vi "Divide Sweep Config by Output Gain.vi"(8 "error in (no error)":errorcluster, 11 "Instrument.DAQ":refnum<class "Instrument.DAQ.lvclass">) -> (0 "error out":errorcluster, 3 "Instrument.DAQ out":refnum<class "Instrument.DAQ.lvclass">)   [LabVIEW 2019, in "Instrument.Lockin.lvlib" / "Instrument.DAQ.lvclass"]
uses:
  Instrument.DAQ.lvclass
  Instrument.DAQ.lvclass/Instrument.DAQ.ctl
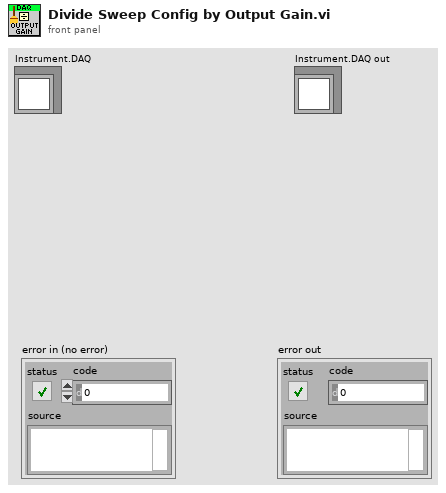
[diagram p1: front panel]
types:
  T1 = typedef "Instrument.Lockin.lvlib/Instrument.DAQ.lvclass/Sweep.Channel--Cluster--Array.ctl" = T2[]
  T2 = typedef "Instrument.Lockin.lvlib/Instrument.DAQ.lvclass/Sweep.Channel--Cluster.ctl" = cluster{"Enable?":bool, "Channel":u16, "Start":dbl, "End":dbl, "Pattern":T3, "Table":dbl[]}
  T3 = typedef "Instrument.Lockin.lvlib/Instrument.DAQ.lvclass/Sweep.Pattern--Enum.ctl" = enum16{"Ramp /", "Ramp /\\", "Smooth Ramp _/", "Smooth Ramp _/\\_", "Table"}
  T4 = typedef "Instrument.Lockin.lvlib/Instrument.DAQ.lvclass/Channel.Gain--Cluster--Array.ctl" = T5[]
  T5 = typedef "Instrument.Lockin.lvlib/Instrument.DAQ.lvclass/Channel.Gain--Cluster.ctl" = cluster{"Channel":string, "Gain":dbl}
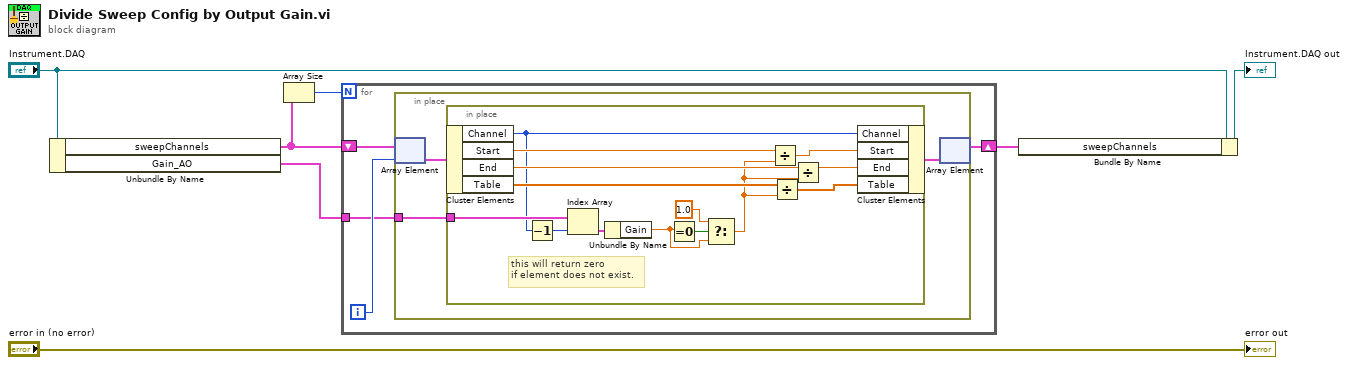
[diagram p0: block diagram]
diagram:
  n1 = Unbundle By Name("Instrument.DAQ") -> ("sweepChannels"=w5:T1, "Gain_AO"=w1:T4)
  n2 = Array Size(array=w5) -> (size(s)=w6:i32)
  n3 = for {
    N: w6 -> [_]
    tunnel: w1 -> [w8]
    shift-right: [w11] -> w2
    shift-left: w5 -> [w9]
    i -> [w10]
    n4 = in-place {
      in-place-border: w8 -> [w12]
      n5 = in-place-array #1(w9, w10) -> (w13:T2)
      n6 = in-place {
        in-place-border: w12 -> [w19]
        # "this will return zero\nif element does not exist."
        n7 = in-place-cluster #2(w13) -> ("Channel"=w16:u16, "Start"=w28:dbl, "End"=w26:dbl, "Table"=w24:dbl[])
        n8 = Decrement(x=w16) -> (x-1=w17:u16)
        n9 = Index Array(array=w19, index=w17) -> (element=w21:T5)
        n10 = Unbundle By Name(w21) -> ("Gain"=w22:dbl)
        n11 = Equal To 0?(x=w22) -> (x = 0?=w20:bool)
        n12 = Select(t=1.0, s=w20, f=w22) -> (s? t:f=w18:dbl)
        n13 = Divide(x=w28, y=w18) -> (x/y=w27:dbl)
        n14 = Divide(x=w24, y=w18) -> (x/y=w23:dbl[])
        n15 = Divide(x=w26, y=w18) -> (x/y=w25:dbl)
        n16 = in-place-cluster #2("Channel"=w16, "Start"=w27, "End"=w25, "Table"=w23) -> (w14:T2)
      }
      n17 = in-place-array #1(w14) -> (w11:T1)  [unwired: 1 out]
    }
  }
  n18 = Bundle By Name(cluster="Instrument.DAQ", "sweepChannels"=w2) -> (→"Instrument.DAQ out":refnum<class "Instrument.DAQ.lvclass">)
  "error out" <- "error in (no error)"
